vi "Create StringMessage.vi"(8 "error in (no error)":errorcluster, 10 "Message Data":string, 11 "Message Name":string) -> (0 "error out":errorcluster, 3 "StringMsg out":refnum<class "StringMessage.lvclass">)   [LabVIEW 2009, in "LapDog.Messaging.v2.NativeTypes.lvlib" / "StringMessage.lvclass"]
doc: "Returns a StringMessage object with the given name."
uses:
  StringMessage.lvclass
  StringMessage.lvclass/StringMessage.ctl
  Messaging.v2/MessageObject/Message.lvclass
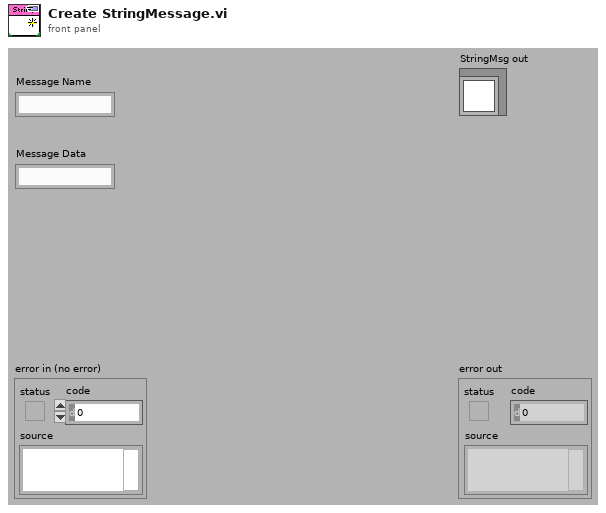
[diagram p1: front panel]
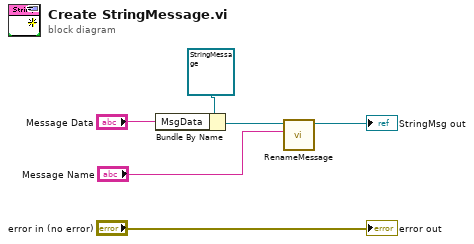
[diagram p0: block diagram]
diagram:
  n1 = Bundle By Name(cluster=refnum<class "StringMessage.lvclass"> refnum ("StringMsg in"), "MsgData"="Message Data") -> (w4:refnum<class "StringMessage.lvclass">)
  n2 = call "RenameMessage.vi"("Message Name"="Message Name", "Message in"=w4) -> ("Message out"=→"StringMsg out":refnum<class "StringMessage.lvclass">)  [unwired: 8 in, 1 out]
  "error out" <- "error in (no error)"
